vi "Saturation (DBL Array).vi"(2 "lower limit":dbl format="%.2f", 3 "upper limit":dbl format="%.2f", 4 "Input Points":dbl[](array[numeric]) format="%.2f") -> (1 "Output Points":dbl[](array[numeric]) format="%.2f")   [LabVIEW 2017, in "NI_AdvCtrl_nonlinear.lvlib"]
doc: "LabVIEW no longer supports this VI. You can obtain similar functionality by installing the LabVIEW Simulation Module.\n\nLimits the valid range of a signal. The output is equal to the upper limit, if input>upper limit. The output is equal to the lower limit, if input<lower limit. In all other cases it is output=input."
uses:
  <vilib>/addons/control/advanced/NI_AdvCtrl_nonlinear.lvlib
  <vilib>/addons/control/advanced/NI_AdvCtrl_continuous linear.lvlib
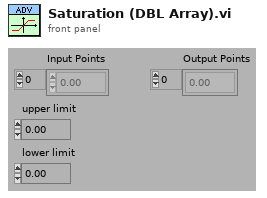
[diagram p1: front panel]
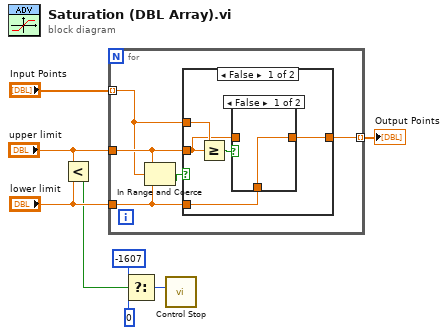
[diagram p0: block diagram]
diagram:
  n1 = Less?(x="upper limit", y="lower limit") -> (x < y?=w2:bool)
  n2 = for {
    tunnel: "lower limit" -> [w13]
    tunnel: "upper limit" -> [w12]
    tunnel: "Input Points" -> [w10] mode=indexing
    tunnel: [w9] -> w5 mode=indexing
    n3 = In Range and Coerce(upper limit=w12, x=w10, lower limit=w13) -> (In Range?=w11:bool)  [unwired: 1 out]
    n4 = case shown="False" w11 {
      tunnel: w10 -> [w18 w21]
      tunnel: [w15 w21] -> w9
      tunnel: w12 -> [w16 _]
      tunnel: w13 -> [w14 _]
      frame False {
        n5 = Greater Or Equal?(x=w18, y=w16) -> (x >= y?=w17:bool)
        n6 = case shown="False" w17 {
          tunnel: w16 -> [_ w20]
          tunnel: [w19 w20] -> w15
          tunnel: w14 -> [w19 _]
          frame False {
          }
          frame True {
          }
        }
      }
      frame True {
      }
    }
  }
  "Output Points" <- w5
  n7 = Select(t=-1607, s=w2, f=0) -> (s? t:f=w1:i32)
  n8 = call <vilib>:"Control Stop.vi"("error"=w1) -> ()  [unwired: 2 out]
